vi "Agilent SNA Set Start and Stop Frequencies.vi"(4 "Passthrough (T)":bool=TRUE, 6 "Channel":i8=1 min=1 max=99 step=1, 7 "Agilent SNA & SWP":T1, 8 "error in (no error)":errorcluster, 9 "CW? (f)":bool, 10 "Start/Stop Freqs, MHz":cluster{"Fstart":dbl, "Fstop":dbl}, 11 "VISA Resource Names":T2) -> (0 "error out":errorcluster, 3 "dup VISA Resource Names":T2)   [LabVIEW 2011]
doc: "This VI for the HP 8753B is used to read the number of stimulus points."
uses:
  TypeDefs/Agilent SNA VISA.ctl
  TypeDefs/Agilent SNA Instrument Info.ctl
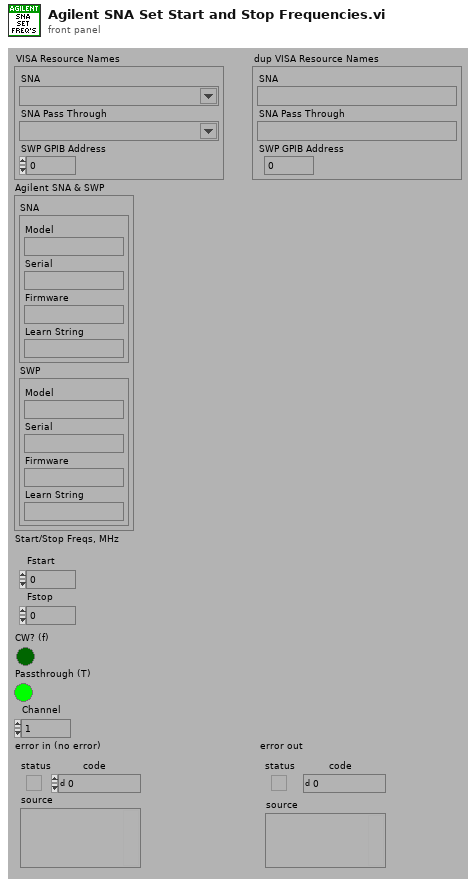
[diagram p1: front panel]
types:
  T1 = typedef "Agilent SNA Instrument Info.ctl" = cluster{"SNA":cluster{"Model":string, "Serial":string, "Firmware":string, "Learn String":string}, "SWP":cluster{"Model":string, "Serial":string, "Firmware":string, "Learn String":string}}
  T2 = typedef "Agilent SNA VISA.ctl" = cluster{"SNA":refnum<visa-resource-name>, "SNA Pass Through":refnum<visa-resource-name>, "SWP GPIB Address":i32}
  T3 = typedef "Agilent SNA Model.ctl" = enum16{"Not Supported", "8757X"}
  T4 = typedef "Agilent SNA SWP Model.ctl" = enum16{"Not Supported", "836XXX", "8375XX", "E82X7D"}
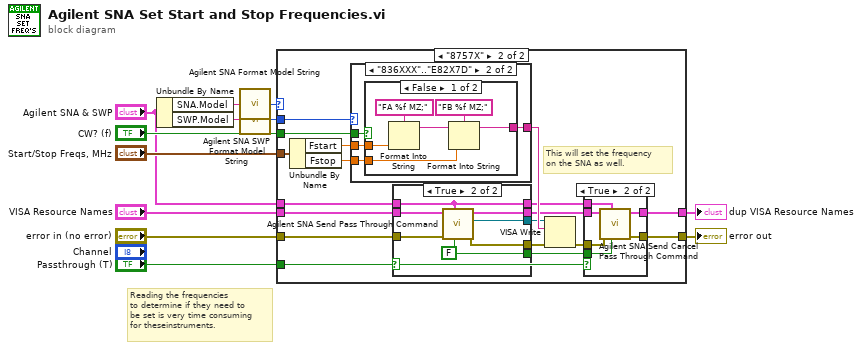
[diagram p0: block diagram]
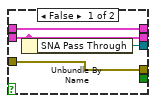
[diagram p4: hidden frame]
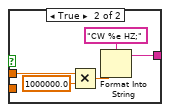
[diagram p6: hidden frame]
diagram:
  # "Reading the frequencies\nto determine if they need to\nbe set is very time consuming\nfor theseinstruments."
  n1 = Unbundle By Name("Agilent SNA & SWP") -> ("SNA.Model"=w9:string, "SWP.Model"=w7:string)
  n2 = call "Agilent SNA Format Model String.vi"("Model String"=w9) -> ("Model"=w8:T3)
  n3 = call "Agilent SNA SWP Format Model String.vi"("Model String"=w7) -> ("Model"=w6:T4)
  n4 = case shown="\"8757X\"" w8 {
    tunnel: [w14 w17] -> w12
    tunnel: "Start/Stop Freqs, MHz" -> [_ w32]
    tunnel: "CW? (f)" -> [_ w31]
    tunnel: "error in (no error)" -> [w14 w24]
    tunnel: "Agilent SNA & SWP" -> [_ w26]
    tunnel: "VISA Resource Names" -> [w13 w25]
    tunnel: w6 -> [_ w27]
    tunnel: [w13 w18] -> w5
    tunnel: "Passthrough (T)" -> [_ w15]
    frame "Not Supported" {
    }
    frame "8757X" {
      # "This will set the frequency\non the SNA as well."
      n5 = Unbundle By Name(w32) -> ("Fstart"=w30:dbl, "Fstop"=w29:dbl)
      n6 = case shown="\"836XXX\"..\"E82X7D\"" w27 {
        tunnel: [_ w55] -> w28
        tunnel: w31 -> [_ w54]
        tunnel: w30 -> [_ w53]
        tunnel: w29 -> [_ w52]
        frame "Not Supported" {
        }
        frame "836XXX".."E82X7D" {
          n7 = case shown="False" w54 {
            tunnel: w53 -> [w59 w65]
            tunnel: w52 -> [w58 _]
            tunnel: [w56 w64] -> w55
            frame False {
              n8 = Format Into String(format string="FA %f MZ;", w59) -> (resulting string=w57:string)  [unwired: 2 in, 1 out]
              n9 = Format Into String(format string="FB %f MZ;", initial string=w57, w58) -> (resulting string=w56:string)  [unwired: 1 in, 1 out]
            }
            frame True {
              n10 = Multiply(x=w65, y=1000000.0) -> (x*y=w62:dbl)
              n11 = Format Into String(format string="CW %e HZ;", w62) -> (resulting string=w64:string)  [unwired: 2 in, 1 out]
            }
          }
        }
      }
      n12 = case shown="True" w15 {
        tunnel: [w42 w51] -> w19
        tunnel: w24 -> [w43 w50]
        tunnel: w25 -> [w41 w49]
        tunnel: [w43 w48] -> w21
        tunnel: w26 -> [w44 w45]
        tunnel: [w41 w47] -> w22
        tunnel: [_ w46] -> w16
        tunnel: [w44 w45] -> w23
        frame False {
          n13 = Unbundle By Name(w41) -> ("SNA Pass Through"=w42:refnum<visa-resource-name>)
        }
        frame True {
          w46 = FALSE ("SCPI? (F)")
          n14 = call "Agilent SNA Send Pass Through Command.vi"("SCPI? (F)"=w46, "Agilent SNA & SWP"=w45, "error in (no error)"=w50, "VISA Resource Names"=w49) -> ("error out"=w48:errorcluster, "SNA Pass Through"=w51:refnum<visa-resource-name>, "dup VISA Resource Names"=w47:T2)  [unwired: 5 out]
        }
      }
      n15 = VISA Write(VISA resource name=w19, write buffer=w28, error in (no error)=w21) -> (error out=w20:errorcluster)  [unwired: 2 out]
      n16 = case shown="True" w15 {
        tunnel: [w34 w40] -> w17
        tunnel: w22 -> [w33 w39]
        tunnel: w20 -> [w34 w38]
        tunnel: w16 -> [_ w37]
        tunnel: [w33 w36] -> w18
        tunnel: w23 -> [_ w35]
        frame False {
        }
        frame True {
          n17 = call "Agilent SNA Send Cancel Pass Through Command.vi"("SCPI? (F)"=w37, "Agilent SNA & SWP"=w35, "error in (no error)"=w38, "VISA Resource Names"=w39) -> ("error out"=w40:errorcluster, "dup VISA Resource Names"=w36:T2)  [unwired: 6 out]
        }
      }
    }
  }
  "dup VISA Resource Names" <- w5
  "error out" <- w12
